vi "subAvi4.vi"(8 "Numeric 4":dbl, 9 "Numeric 3":dbl, 10 "Numeric 2":dbl, 11 "Numeric":dbl) -> (3 "res":dbl)   [LabVIEW 2019]
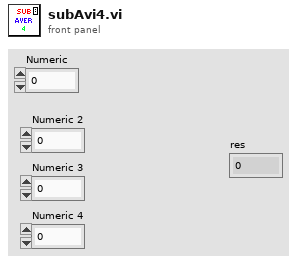
[diagram p1: front panel]
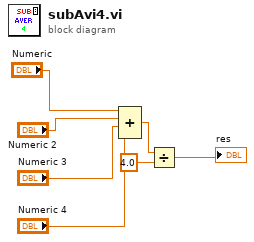
[diagram p0: block diagram]
diagram:
  n1 = Compound Arithmetic op=ADD("Numeric", "Numeric 2", "Numeric 3", "Numeric 4") -> (w3:dbl)
  n2 = Divide(x=w3, y=4.0) -> (x/y=→"res":dbl)
